vi "insert string&image into excel.vi"(8 "error in":errorcluster, 10 "Item_Information":T1, 11 "template Path":path) -> (0 "error out":errorcluster, 3 "report out":refnum<class "NI_report.lvclass">)   [LabVIEW 2017]
doc: "This program is used to insert string and QR code to excel. To print label for ASTI's factory.\nUser enters Cluster string(Item Information). Program will be automatically exported excel file."
uses:
  Control/Label data.ctl
  <vilib>/Utility/NIReport.llb/NI_report.lvclass
  QR Code Generator v1.1.llb/User Option.ctl
  QR Code Generator v1.1.llb/EC Level.ctl
  <vilib>/picture/picture.llb/Draw 1-Bit Pixmap.vi
  <vilib>/addons/_office/NI_ReportGenerationToolkit.lvlib
  <vilib>/Utility/NIReport.llb/Excel/NI_Excel.lvclass
panel:
  out "QR Code":picture
  out "Area Draw":cluster{dbl, dbl}
  out "QR Size":i32
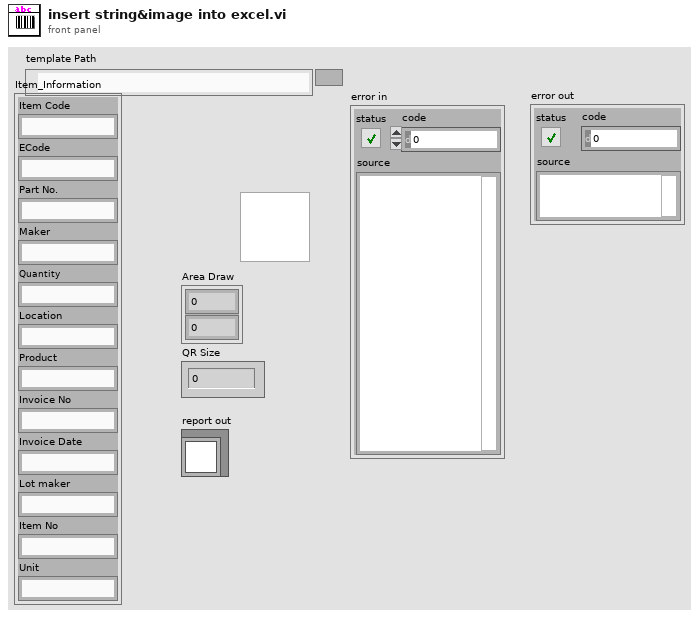
[diagram p1: front panel]
types:
  T1 = typedef "Label data.ctl" = cluster{"Item Code":string, "ECode":string, "Part No.":string, "Maker":string, "Quantity":string, "Location":string, "Product":string, "Invoice No":string, "Invoice Date":string, "Lot maker":string, "Item No":string, "Unit":string}
  T2 = enum16{"maximized", "minimized", "normal", "no change"}
  T3 = enum16{"Standard Report", "HTML", "Word", "Excel"}
  T4 = typedef "EC Level.ctl" = enum16{"L", "M", "Q", "H"}
  T5 = typedef "User Option.ctl" = enum32{"Automatic", "Numeric", "Alphanumeric", "Plain Text / Website", "Contact Number", "Email Address", "SMS Message"}
  T6 = cluster{"position (Excel)":cluster{"row":i32, "column":i32}, "name (Excel)":string, "bookmark (Word)":string}
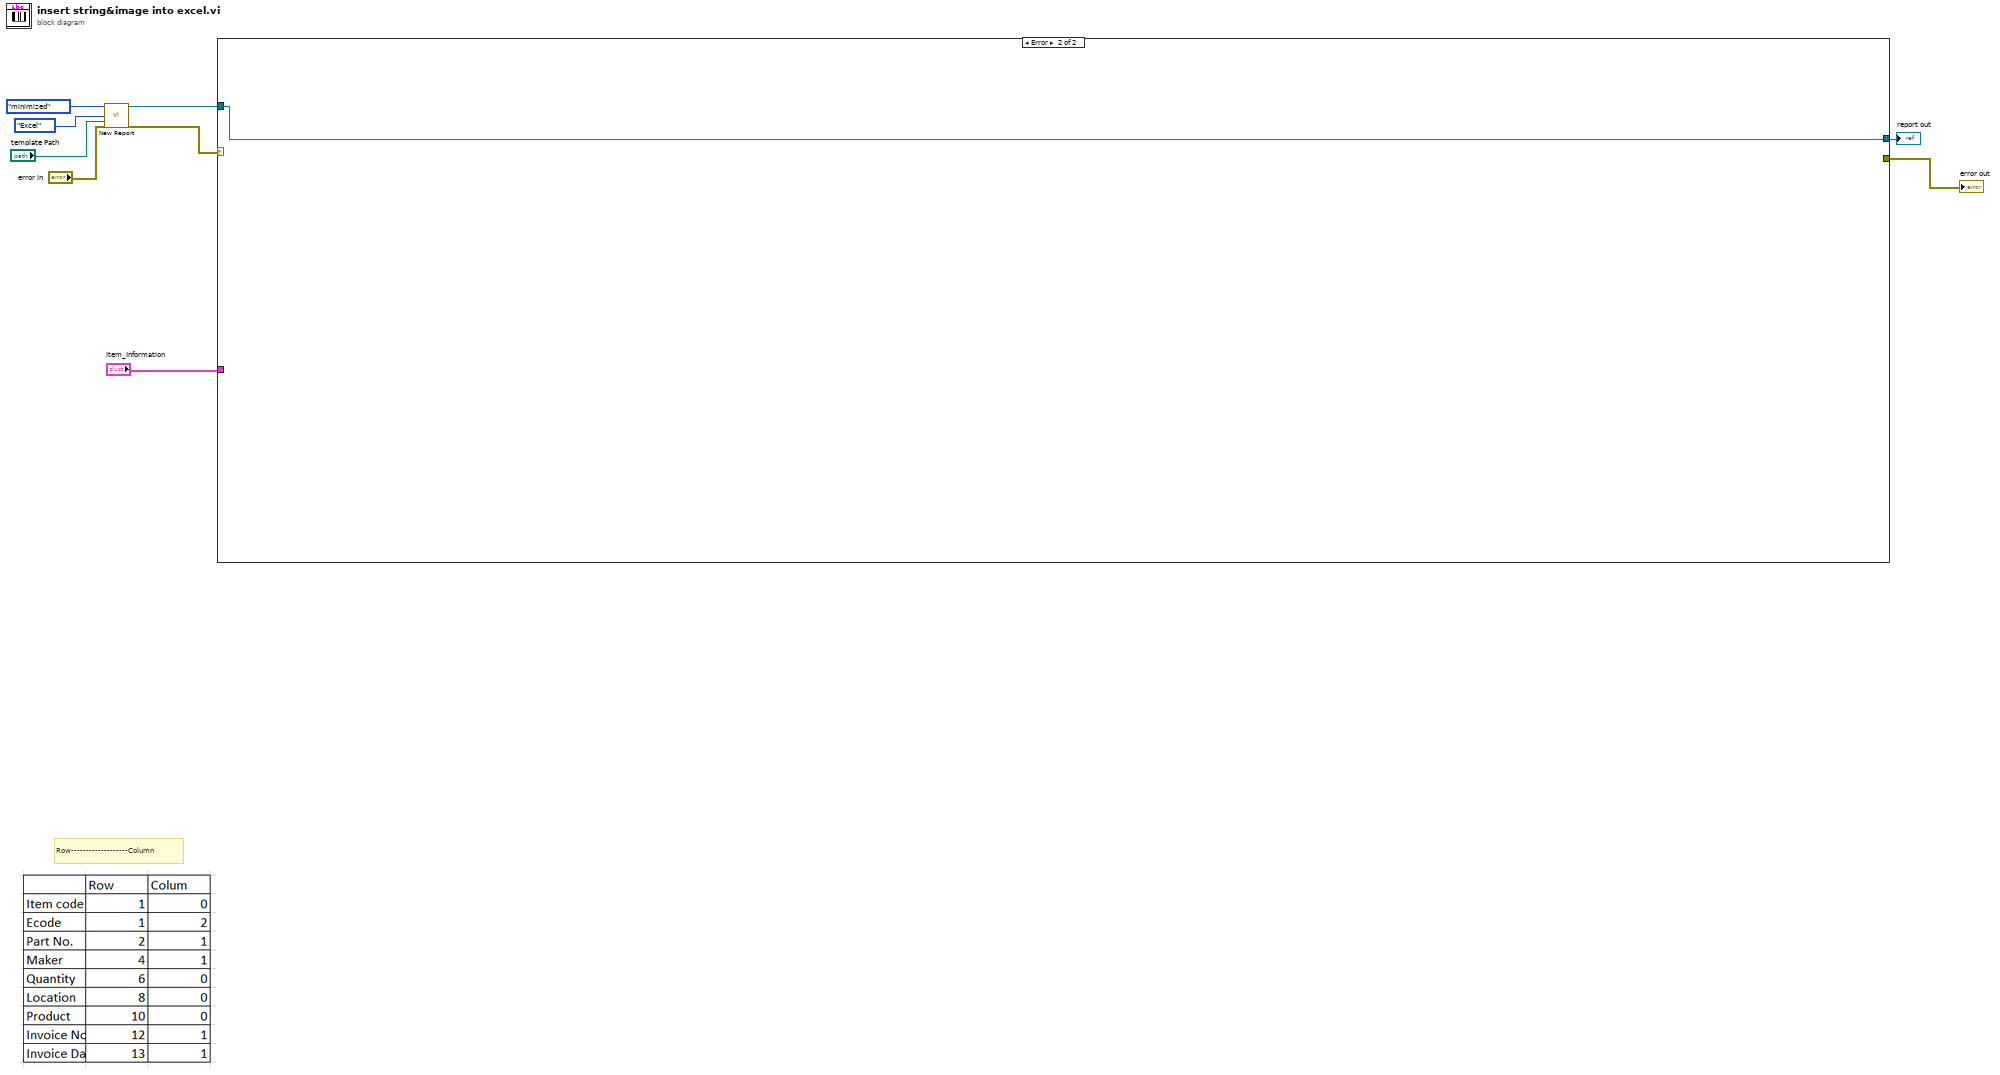
[diagram p0: block diagram]
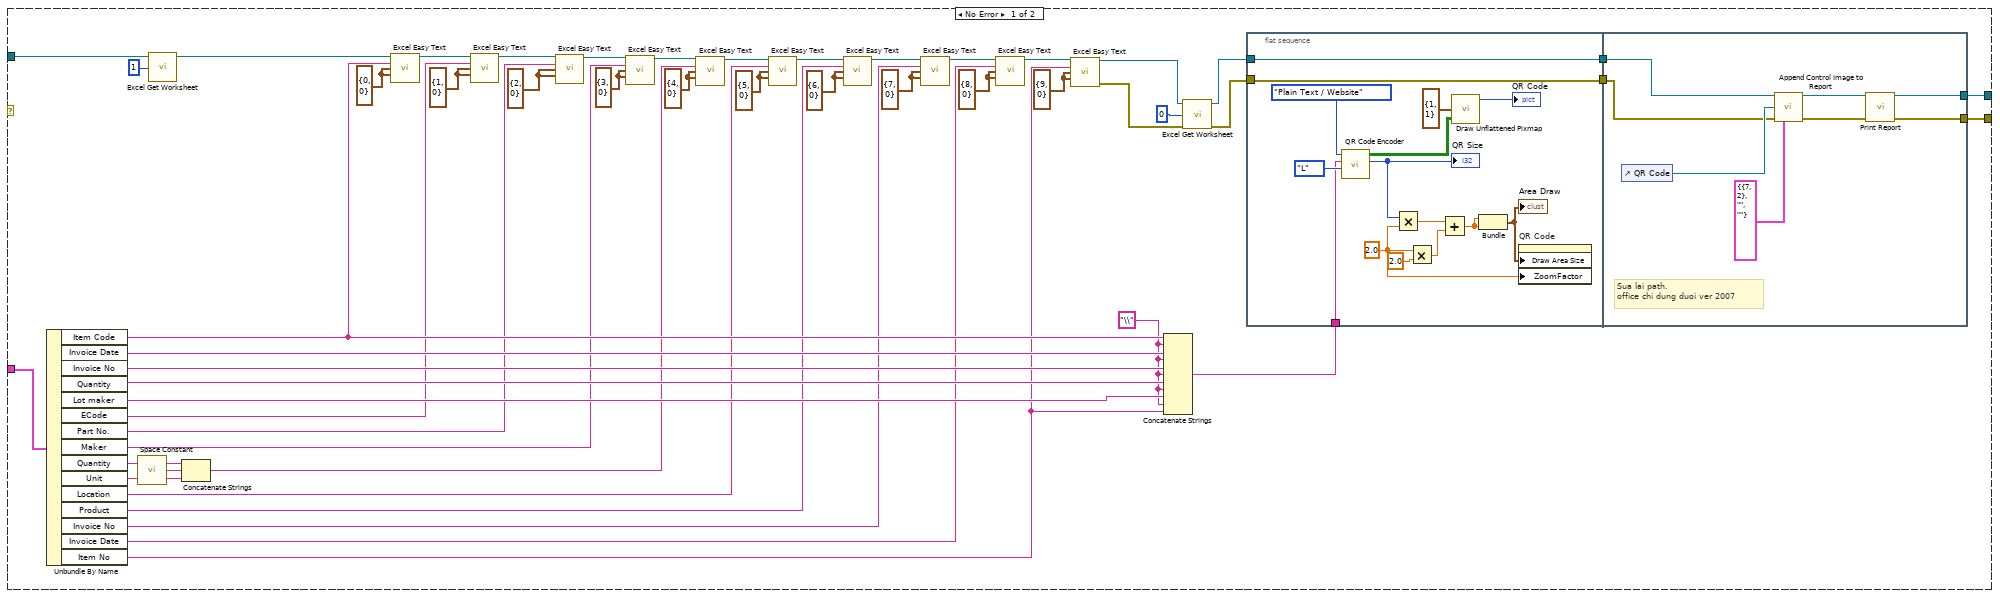
[diagram p2: hidden frame]
diagram:
  # "Row-------------------Column"
  n1 = call <vilib>:"New Report.vi"("window state (normal)"=T2."minimized", "report type"=T3."Excel", "template (empty)"="template Path", "error in (no error)"="error in") -> ("report out"=w5:refnum<class "NI_report.lvclass">, "error out"=w3:errorcluster)  [unwired: 10 in]
  n2 = case shown="Error" w3 {
    tunnel: [w60 _] -> w9
    tunnel: "Item_Information" -> [w59 _]
    tunnel: w5 -> [w20 w84]
    tunnel: [w12 w84] -> w1
    frame No Error {
      w22 = cluster{"row":i32, "column":i32} {"row"=9, "column"=0} ("start (-1, -1)")
      w26 = cluster{"row":i32, "column":i32} {"row"=8, "column"=0} ("start (-1, -1)")
      w29 = cluster{"row":i32, "column":i32} {"row"=7, "column"=0} ("start (-1, -1)")
      w32 = cluster{"row":i32, "column":i32} {"row"=6, "column"=0} ("start (-1, -1)")
      w35 = cluster{"row":i32, "column":i32} {"row"=5, "column"=0} ("start (-1, -1)")
      w38 = cluster{"row":i32, "column":i32} {"row"=4, "column"=0} ("start (-1, -1)")
      w44 = cluster{"row":i32, "column":i32} {"row"=3, "column"=0} ("start (-1, -1)")
      w47 = cluster{"row":i32, "column":i32} {"row"=2, "column"=0} ("start (-1, -1)")
      w50 = cluster{"row":i32, "column":i32} {"row"=1, "column"=0} ("start (-1, -1)")
      w52 = cluster{"row":i32, "column":i32} {"row"=0, "column"=0} ("start (-1, -1)")
      w11 = "\\" ("string")
      n3 = Unbundle By Name(w59) -> ("Item Code"=w53:string, "Invoice Date"=w58:string, "Invoice No"=w57:string, "Quantity"=w56:string, "Lot maker"=w55:string, "ECode"=w51:string, "Part No."=w48:string, "Maker"=w45:string, "Quantity"=w42:string, "Unit"=w40:string, "Location"=w36:string, "Product"=w33:string, "Invoice No"=w30:string, "Invoice Date"=w27:string, "Item No"=w10:string)
      n4 = call <vilib>:"Space Constant.vi"() -> ("String"=w41:string)
      n5 = call <vilib>:"Excel Get Worksheet.vi"("report in"=w20, "worksheet index (0)"=1) -> ("report out"=w19:refnum<class "NI_report.lvclass">)  [unwired: 12 in, 1 out]
      n6 = Concatenate Strings(w42, w41, w40) -> (w39:string)
      n7 = call <vilib>:"Excel Easy Text.vi"("report in"=w19, "text"=w53, "start (-1, -1)"=w52, "end (-1, -1)"=w52) -> ("report out"=w21:refnum<class "NI_report.lvclass">)  [unwired: 7 in, 4 out]
      n8 = call <vilib>:"Excel Easy Text.vi"("report in"=w21, "text"=w51, "start (-1, -1)"=w50, "end (-1, -1)"=w50) -> ("report out"=w49:refnum<class "NI_report.lvclass">)  [unwired: 7 in, 4 out]
      n9 = call <vilib>:"Excel Easy Text.vi"("report in"=w49, "text"=w48, "start (-1, -1)"=w47, "end (-1, -1)"=w47) -> ("report out"=w46:refnum<class "NI_report.lvclass">)  [unwired: 7 in, 4 out]
      n10 = call <vilib>:"Excel Easy Text.vi"("report in"=w46, "text"=w45, "start (-1, -1)"=w44, "end (-1, -1)"=w44) -> ("report out"=w43:refnum<class "NI_report.lvclass">)  [unwired: 7 in, 4 out]
      n11 = call <vilib>:"Excel Easy Text.vi"("report in"=w43, "text"=w39, "start (-1, -1)"=w38, "end (-1, -1)"=w38) -> ("report out"=w37:refnum<class "NI_report.lvclass">)  [unwired: 7 in, 4 out]
      n12 = call <vilib>:"Excel Easy Text.vi"("report in"=w37, "text"=w36, "start (-1, -1)"=w35, "end (-1, -1)"=w35) -> ("report out"=w34:refnum<class "NI_report.lvclass">)  [unwired: 7 in, 4 out]
      n13 = call <vilib>:"Excel Easy Text.vi"("report in"=w34, "text"=w33, "start (-1, -1)"=w32, "end (-1, -1)"=w32) -> ("report out"=w31:refnum<class "NI_report.lvclass">)  [unwired: 7 in, 4 out]
      n14 = call <vilib>:"Excel Easy Text.vi"("report in"=w31, "text"=w30, "start (-1, -1)"=w29, "end (-1, -1)"=w29) -> ("report out"=w28:refnum<class "NI_report.lvclass">)  [unwired: 7 in, 4 out]
      n15 = call <vilib>:"Excel Easy Text.vi"("report in"=w28, "text"=w27, "start (-1, -1)"=w26, "end (-1, -1)"=w26) -> ("report out"=w23:refnum<class "NI_report.lvclass">)  [unwired: 7 in, 4 out]
      n16 = call <vilib>:"Excel Easy Text.vi"("report in"=w23, "text"=w10, "start (-1, -1)"=w22, "end (-1, -1)"=w22) -> ("report out"=w16:refnum<class "NI_report.lvclass">, "error out"=w13:errorcluster)  [unwired: 7 in, 3 out]
      n17 = Concatenate Strings(w53, w11, w58, w11, w57, w11, w56, w11, w55, w11, w10) -> (w54:string)
      n18 = call <vilib>:"Excel Get Worksheet.vi"("report in"=w16, "worksheet index (0)"=0, "error in (no error)"=w13) -> ("report out"=w15:refnum<class "NI_report.lvclass">, "error out"=w14:errorcluster)  [unwired: 11 in]
      n19 = flat-sequence {
        tunnel: [w63] -> w25
        tunnel: w14 -> [w63]
        tunnel: w54 -> [w62]
        tunnel: [w61] -> w24
        tunnel: w15 -> [w61]
        tunnel: [w78] -> w60
        tunnel: w25 -> [w80]
        tunnel: w24 -> [w79]
        tunnel: [w76] -> w12
        frame #0 {
          w65 = 2.0 ("size")
          n20 = call "QR Code Encoder.vi"("EC Level"=EC_Level."L", "Message"=w62, "User Option"=User_Option."Plain Text / Website") -> ("QR Size"=w66:i32, "QR Data"=w73:bool[][])  [unwired: 7 in]
          "QR Size" <- w66
          n21 = Multiply(x=w66, y=w65) -> (x*y=w64:dbl)
          n22 = Multiply(x=w65, y=2.0) -> (x*y=w68:dbl)
          n23 = Add(x=w64, y=w68) -> (x+y=w67:dbl)
          n24 = call-poly <vilib>:"Draw Unflattened Pixmap.vi"("top left point(0, 0)"=cluster{"x":i16, "y":i16} {"x"=1, "y"=1}, "data"=w73) -> ("new picture"=→"QR Code":picture)  [unwired: 7 in]
          n25 = Bundle(w67, w67) -> (w70:cluster{dbl, dbl})  [unwired: 1 in]
          "Area Draw" <- w70
          n26 = property on="QR Code" class="Pict"("Draw Area Size"=w70, "ZoomFactor"=w65) -> ()  [unwired: 2 in, 2 out]
        }
        frame #1 {
          # "Sua lai path.\noffice chi dung duoi ver 2007"
          n27 = control-ref of="QR Code"() -> (w83:refnum<vi>)
          n28 = call-dynamic "Append Control Image to Report.vi"("report in"=w79, "ctrl reference"=w83, "error in (no error)"=w80, "MS Office parameters"=T6 {"position (Excel)"={"row"=7, "column"=2}, "name (Excel)"="", "bookmark (Word)"=""}) -> ("report out"=w77:refnum<class "NI_report.lvclass">, "error out"=w81:errorcluster)  [unwired: 8 in, 2 out]
          n29 = call-dynamic "Print Report.vi"("report in"=w77, "error in (no error)"=w81) -> ("report out"=w76:refnum<class "NI_report.lvclass">, "error out"=w78:errorcluster)  [unwired: 12 in]
        }
      }
    }
    frame Error {
    }
  }
  "error out" <- w9
  "report out" <- w1
